vi "testVI.vi"() -> ()   [LabVIEW 2010]
uses:
  <vilib>/Utility/inputDevices.llb/closeJoystick.vi
  C:/Documents and Settings/hakonnod/Desktop/Rotate.llb/rotate 24bit.vi
  <vilib>/picture/picture.llb/Draw True-Color Pixmap.vi
  <vilib>/Utility/inputDevices.llb/joystickAcquire.vi
  <vilib>/picture/3D Picture Control/NI_3D Picture Control.lvlib
panel:
  out "Dial 2":dbl
  in  "Dial":dbl(knob)=4.820308593039098 scale=0.0..10.0
  out "Picture 2":picture
  in  "stop 3":bool
  in  "Pen Color":u32(colorbox)=15671808
  in  "Line Marker":T1={"Width"=1, "Style"=enum."Solid"}
  in  "Rotation Angle (degrees)":dbl=30.0 format="%.2f"
  out "Numeric 5":dbl
  out "Numeric 3":dbl
  out "Numeric 2":dbl
  out "Joystick Info":T2(array[cluster])
  out "Numeric":dbl
  in  "stop 2":bool
  out "Picture":picture
  in  "stop":bool
  out "3D Picture":refnum<vi>(3d-picture)
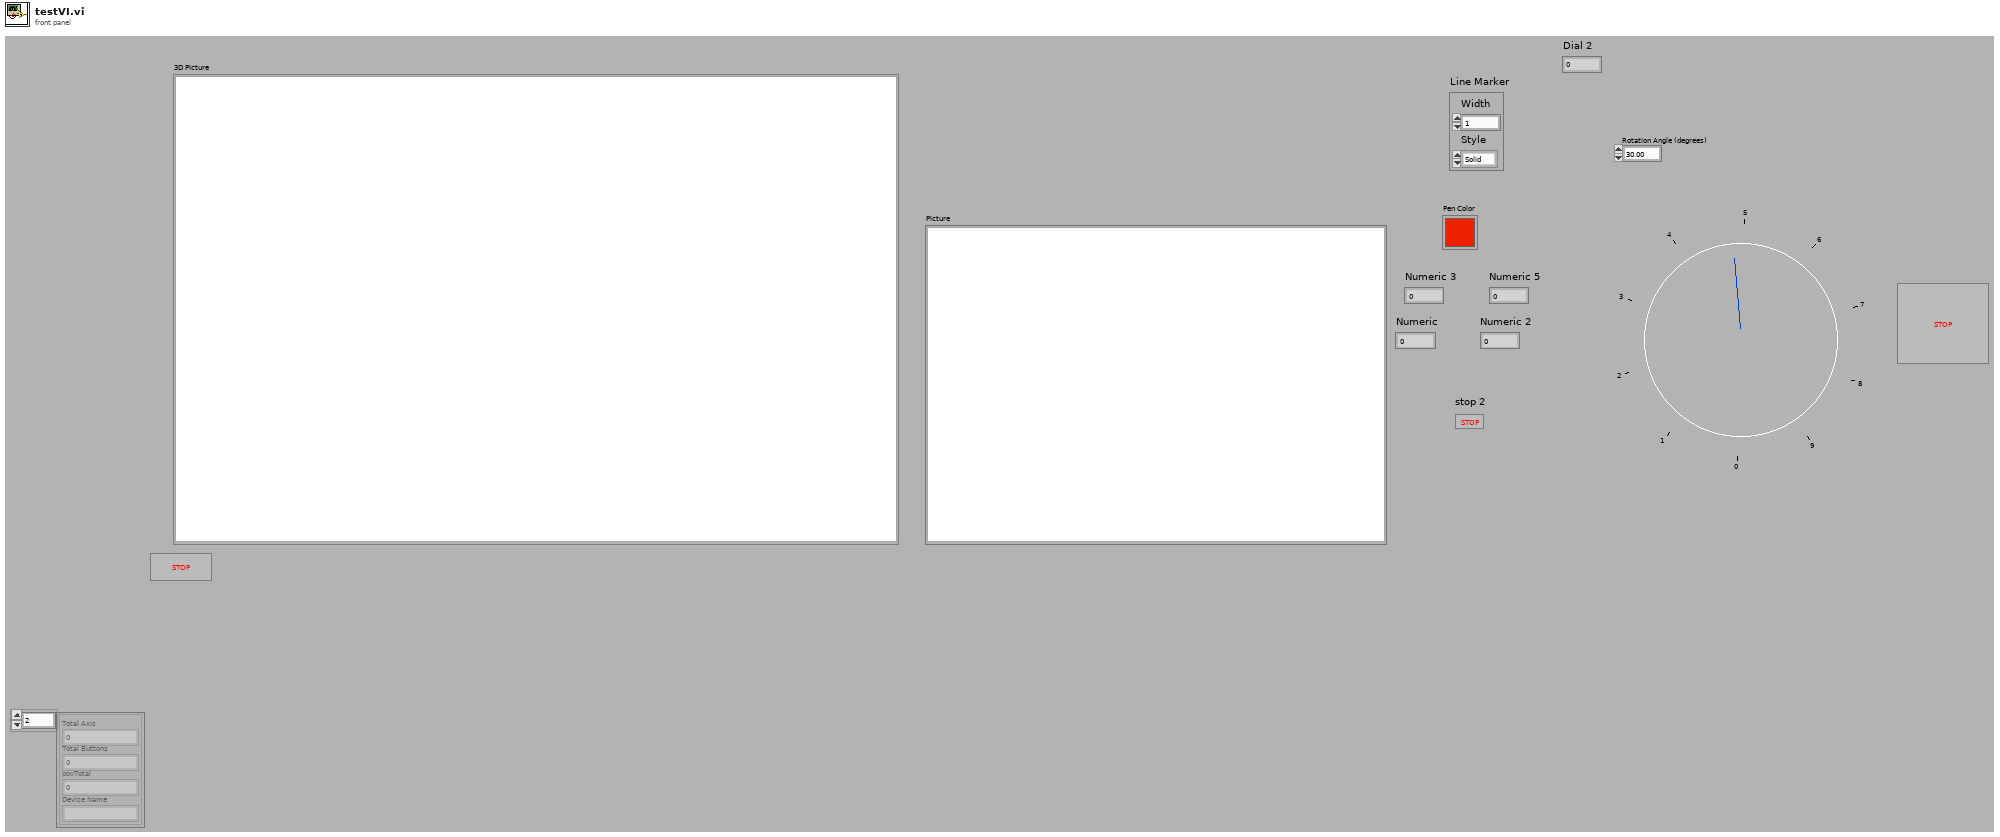
[diagram p1: front panel]
types:
  T1 = cluster{"Width":u16, "Style":enum32{"Solid", "Dash", "Dot", "DashDot", "DashDotDot"}}
  T2 = cluster{"Total Axis":u32, "Total Buttons":u32, "povTotal":u32, "Device Name":string}[]
  T3 = cluster{"Red":sgl, "Green":sgl, "Blue":sgl, "Alpha":sgl}
  T4 = cluster{"axes total":u32, "buttons total":u32, "pov total":u32, "device name":string}[]
  T5 = cluster{"X axis":i32, "Y axis":i32, "Z axis":i32, "X axis rotation":i32, "Y axis rotation":i32, "Z axis rotation":i32, "U axis":i32, "V axis":i32}
  T6 = typedef "imagedata.ctl" = cluster{"image type":i32, "image depth":i32, "image":u8[], "mask":u8[], "colors":u32[], "Rectangle":cluster{"left":i16, "top":i16, "right":i16, "bottom":i16}}
  T7 = typedef "LVMouseTypeDef.ctl" = cluster{"Mouse Position":cluster{"X":i32, "Y":i32}, "Mouse Modifiers":cluster{"Button Down":bool, "Shift Mod":bool, "Menu Mod":bool, "Option Mod":bool}}
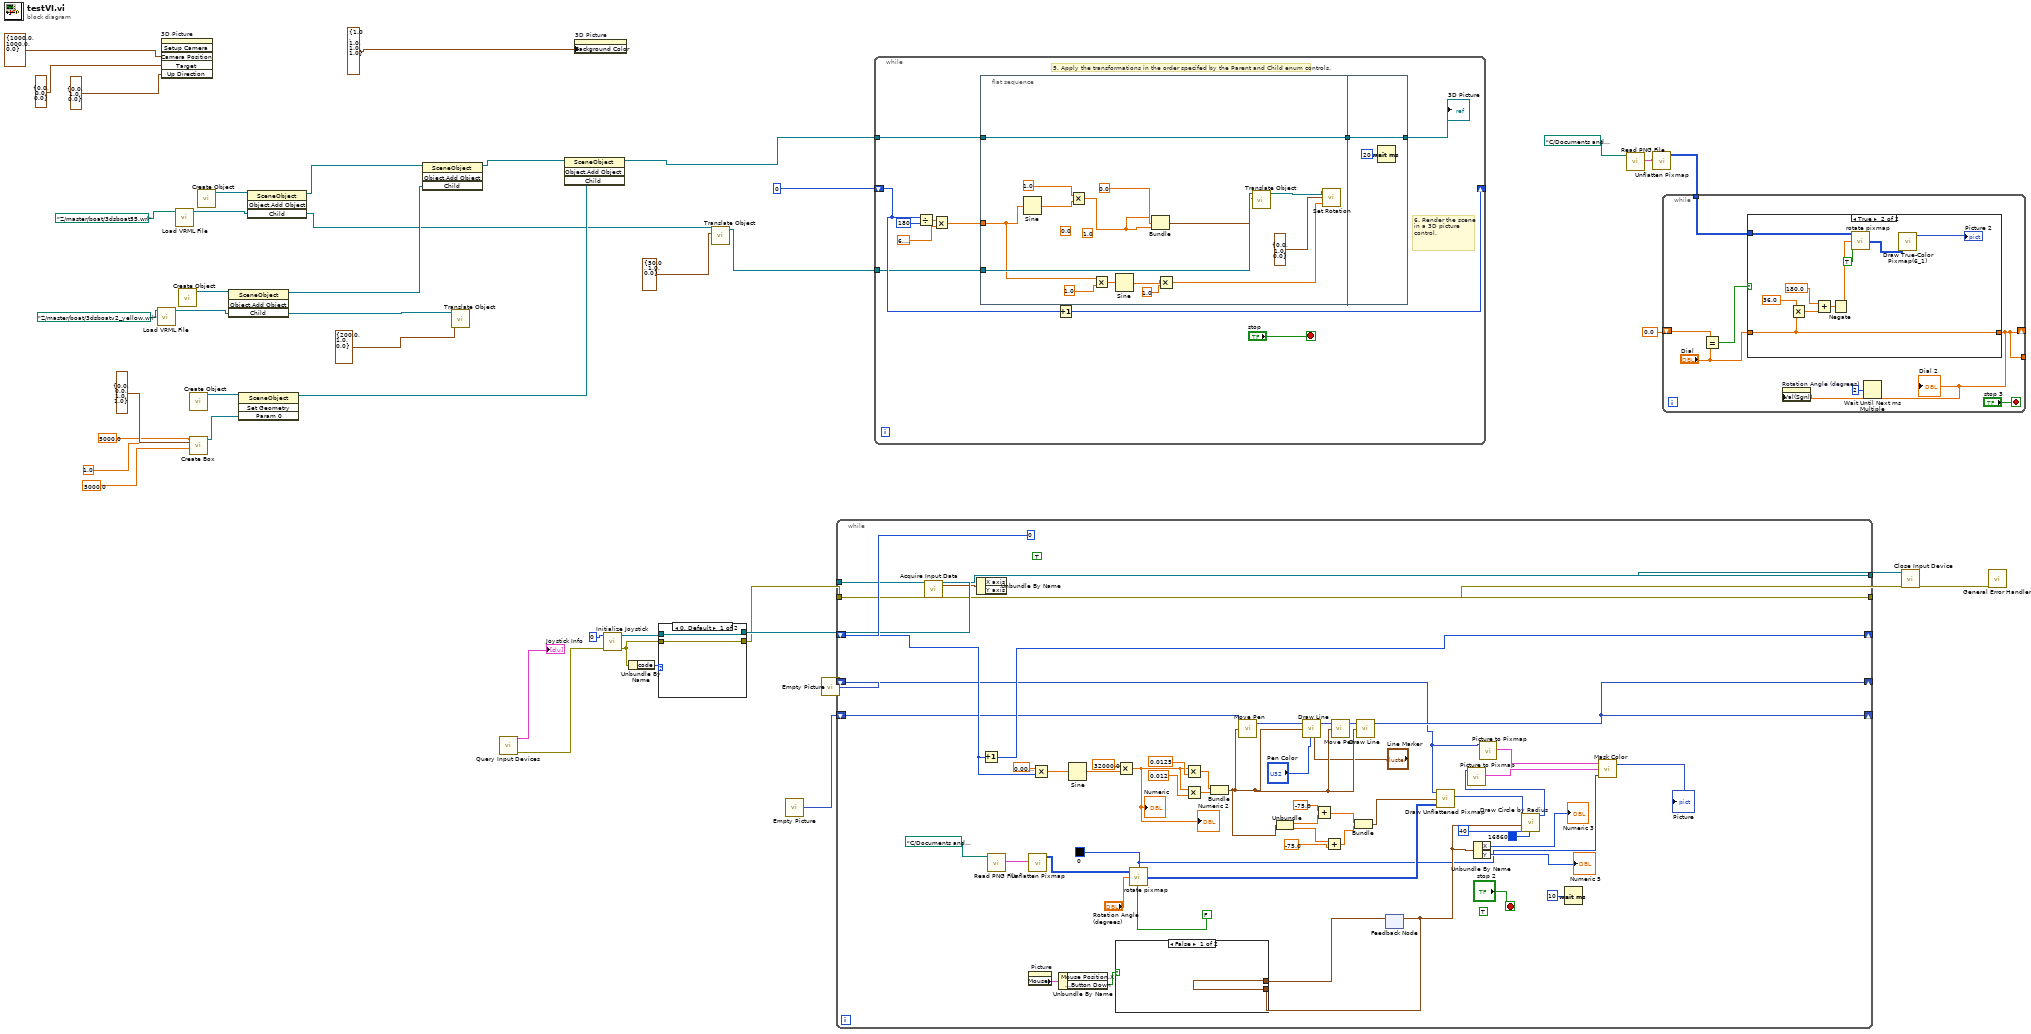
[diagram p0: block diagram]
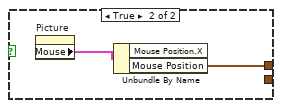
[diagram p4: hidden frame]
diagram:
  (unwired) TRUE
  n1 = call <vilib>:"Load VRML File.vi"("Path"=path "Z:/master/boat/3dsboatv2_yellow.wrl") -> ("Scene:Read Scene File"=w25:refnum<vi>)  [unwired: 9 in, 1 out]
  n2 = invoke on="3D Picture" class="SceneGraphDisp (strict)" method="Setup Camera"("Camera Position"=cluster{"X":sgl, "Y":sgl, "Z":sgl} {"X"=1000.0, "Y"=1000.0, "Z"=0.0}, "Target"=cluster{"X":sgl, "Y":sgl, "Z":sgl} {"X"=0.0, "Y"=0.0, "Z"=0.0} ("Camera Position"), "Up Direction"=cluster{"X":sgl, "Y":sgl, "Z":sgl} {"X"=0.0, "Y"=1.0, "Z"=0.0} ("Camera Position")) -> ()  [unwired: 3 in, 6 out]
  n3 = call <vilib>:"Load VRML File.vi"("Path"=path "Z:/master/boat/3dsboat55.wrl") -> ("Scene:Read Scene File"=w36:refnum<vi>)  [unwired: 9 in, 1 out]
  n4 = call <vilib>:"Create Object.vi"() -> ("Scene:New Object"=w26:refnum<vi>)  [unwired: 10 in, 1 out]
  n5 = call <vilib>:"Create Object.vi"() -> ("Scene:New Object"=w41:refnum<vi>)  [unwired: 10 in, 1 out]
  n6 = call <vilib>:"Create Box.vi"("Color"=T3 {"Red"=0.0, "Green"=0.0, "Blue"=1.0, "Alpha"=1.0}, "Length Z"=sgl 5000.0 ("Red"), "Length Y"=sgl 1.0 ("Red"), "Length X"=sgl 5000.0 ("Red")) -> ("New Box Refnum"=w40:refnum<vi>)  [unwired: 6 in, 1 out]
  n7 = call <vilib>:"Create Object.vi"() -> ("Scene:New Object"=w37:refnum<vi>)  [unwired: 10 in, 1 out]
  n8 = invoke class="SceneObject" method="Object.Add Object"(reference=w26, "Child"=w25) -> (reference out=w20:refnum<vi>, "Child"=w24:refnum<vi>)  [unwired: 2 in, 2 out]
  n9 = invoke class="SceneObject" method="Set Geometry"(reference=w41, "Param 0"=w40) -> (reference out=w28:refnum<vi>)  [unwired: 2 in, 3 out]
  n10 = invoke class="SceneObject" method="Object.Add Object"(reference=w37, "Child"=w36) -> (reference out=w22:refnum<vi>, "Child"=w6:refnum<vi>)  [unwired: 2 in, 2 out]
  n11 = invoke class="SceneObject" method="Object.Add Object"(reference=w22, "Child"=w20) -> (reference out=w21:refnum<vi>)  [unwired: 2 in, 3 out]
  n12 = call <vilib>:"Translate Object.vi"("Translation"=cluster{"X":sgl, "Y":sgl, "Z":sgl} {"X"=200.0, "Y"=1.0, "Z"=0.0} ("Camera Position"), "Scene.Object In"=w24) -> ()  [unwired: 8 in, 2 out]
  n13 = call <vilib>:"Query Input Devices.vi"() -> ("error out"=w18:errorcluster, "joystick info"=→"Joystick Info":T4)  [unwired: 1 in, 9 out]
  n14 = invoke class="SceneObject" method="Object.Add Object"(reference=w21, "Child"=w28) -> (reference out=w29:refnum<vi>)  [unwired: 2 in, 3 out]
  n15 = property on="3D Picture" class="SceneGraphDisp (strict)"("Background Color"=cluster{"X":sgl, "Y":sgl, "Z":sgl, "Z 2":sgl} {"X"=1.0, "Y"=1.0, "Z"=1.0, "Z 2"=1.0} ("Camera Position")) -> ()  [unwired: 2 in, 2 out]
  n16 = call <vilib>:"Initialize Joystick.vi"("error in (no error)"=w18, "device index"=0) -> ("error out"=w13:errorcluster, "device ID"=w14:refnum<k1>)  [unwired: 8 out]
  n17 = Unbundle By Name(w13) -> ("code"=w15:i32)
  n18 = case shown="0, Default" w15 {
    tunnel: w13 -> [w47 w49]
    tunnel: [w47 w49] -> w11
    tunnel: w14 -> [w46 w48]
    tunnel: [w46 w48] -> w12
    frame 0, Default {
    }
    frame -2000000008 {
    }
  }
  n19 = call <vilib>:"Translate Object.vi"("Translation"=cluster{"X":sgl, "Y":sgl, "Z":sgl} {"X"=50.0, "Y"=1.0, "Z"=0.0} ("Camera Position"), "Scene.Object In"=w6) -> ("Scene.Object Out"=w31:refnum<vi>)  [unwired: 8 in, 1 out]
  n20 = call "Empty Picture"() -> ("empty picture"=w5:picture)
  n21 = call "Empty Picture"() -> ("empty picture"=w7:picture)
  n22 = while {
    shift-right: [w103] -> _
    shift-left: 0 -> [w84]
    tunnel: w12 -> [w101]
    tunnel: w11 -> [w100]
    tunnel: [w99] -> w9
    tunnel: [w98] -> w8
    shift-right: [w79] -> _
    shift-left: w7 -> [w56]
    shift-right: [w79] -> _
    shift-left: w5 -> [w80]
    stop <- "stop 2" stop-if-true
    w52 = u32 0 ("Fill Color")
    (unwired) TRUE
    n23 = call-poly <vilib>:"Acquire Input Data.vi"("device ID"=w101, "error in (no error)"=w100) -> ("device ID"=w99:refnum<k1>, "axis info"=w97:T5, "error out"=w98:errorcluster)  [unwired: 15 out]
    n24 = Unbundle By Name(w97) -> ()  [unwired: 2 out]
    n25 = Increment(x=w84) -> (x+1=w103:i32)
    n26 = call <vilib>:"Read PNG File.vi"("path to PNG file"=path "C:/Documents and Settings/hakonnod/My Documents/MATLAB/manualThrusterControl/boat.png") -> ("image data"=w61:T6)  [unwired: 8 in, 2 out]
    n27 = call <vilib>:"Unflatten Pixmap.vi"("image data"=w61) -> ("24-bit pixmap"=w71:u32[][])  [unwired: 4 in, 6 out]
    n28 = property on="Picture" class="Pict"() -> ("Mouse"=w96:T7)  [unwired: 2 in, 2 out]
    n29 = Multiply(x=sgl 0.01 ("Z"), y=w84) -> (x*y=w85:sgl)
    n30 = Unbundle By Name(w96) -> ("Mouse Modifiers.Button Down"=w77:bool)  [unwired: 1 out]
    n31 = Sine(x=w85) -> (sin(x)=w89:sgl)
    n32 = Multiply(x=sgl 32000.0 ("Z"), y=w89) -> (x*y=w88:sgl)
    "Numeric" <- w88
    "Numeric 2" <- w88
    n33 = call-poly "rotate pixmap.vi"("Color Table Index of Fill Color"=w52, "Maintain Center Position?"=FALSE, "Rotation Angle (degrees)"="Rotation Angle (degrees)", "Pixmap"=w71) -> ("Rotated Pixmap"=w62:u32[][])
    n34 = Multiply(x=w88, y=0.0125) -> (x*y=w92:dbl)
    n35 = Multiply(x=w88, y=0.012) -> (x*y=w94:dbl)
    n36 = Bundle(w92, w94) -> (w69:cluster{dbl, dbl})  [unwired: 1 in]
    n37 = call <vilib>:"Move Pen.vi"("new position"=w69, "picture"=w80) -> ("new picture"=w91:picture)  [unwired: 3 in]
    n38 = Unbundle(w69) -> (w64:dbl, w68:dbl)
    n39 = call <vilib>:"Draw Line.vi"("picture"=w91, "end point"=w69, "color(black)"="Pen Color", "pen"="Line Marker") -> ("new picture"=w81:picture)  [unwired: 5 in]
    n40 = Add(x=sgl -75.0 ("X"), y=w64) -> (x+y=w63:dbl)
    n41 = Add(x=w68, y=sgl -75.0 ("X")) -> (x+y=w67:dbl)
    n42 = call <vilib>:"Move Pen.vi"("new position"=w69, "picture"=w81) -> ("new picture"=w82:picture)  [unwired: 3 in]
    n43 = Bundle(w63, w67) -> (w70:cluster{dbl, dbl})  [unwired: 1 in]
    n44 = call <vilib>:"Draw Line.vi"("picture"=w82, "end point"=w69) -> ("new picture"=w79:picture)  [unwired: 7 in]
    n45 = feedback #1() -> (w75:cluster{"X":i32, "Y":i32})  [unwired: 1 in]
    n46 = case shown="False" w77 {
      tunnel: [w104 w105] -> w76
      tunnel: w75 -> [w104 _]
      frame False {
      }
      frame True {
        n47 = property on="Picture" class="Pict"() -> ("Mouse"=w106:T7)  [unwired: 2 in, 2 out]
        n48 = Unbundle By Name(w106) -> ("Mouse Position"=w105:cluster{"X":i32, "Y":i32})  [unwired: 1 out]
      }
    }
    n49 = feedback-in #1(w76) -> ()
    n50 = call-poly <vilib>:"Draw Unflattened Pixmap.vi"("picture"=w56, "top left point(0, 0)"=w70, "data (RGB format)"=w62) -> ("new picture"=w57:picture)  [unwired: 6 in]
    n51 = Unbundle By Name(w75) -> ("X"=→"Numeric 3":i32, "Y"=→"Numeric 5":i32)
    n52 = call <vilib>:"Picture to Pixmap.vi"("picture"=w56) -> ("image data"=w60:T6)  [unwired: 9 in, 1 out]
    n53 = call <vilib>:"Draw Circle by Radius.vi"("color(black)"=u32 16860, "pixel center"=w75, "radius"=40, "picture"=w57) -> ("new picture"=w58:picture)  [unwired: 7 in]
    n54 = call <vilib>:"Picture to Pixmap.vi"("picture"=w58) -> ("image data"=w59:T6)  [unwired: 9 in, 1 out]
    n55 = Wait (ms)(milliseconds to wait=10) -> ()  [unwired: 1 out]
    n56 = call "Mask Color.vi"("Current Mask Color"=w52, "mask data"=w59, "image data"=w60) -> ("Picture"=→"Picture":picture)  [unwired: 1 in]
  }
  n57 = while {
    tunnel: w29 -> [w113]
    shift-right: [w109] -> _
    shift-left: 0 -> [w110]
    tunnel: w31 -> [w108]
    stop <- "stop" stop-if-true
    # "6. Render the scene in a 3D picture control."
    # "5. Apply the transformations in the order specifed by the Parent and Child enum controls."
    n58 = Divide(x=w110, y=180) -> (x/y=w116:dbl)
    n59 = Multiply(x=w116, y=6.283185307179586) -> (x*y=w107:dbl)
    n60 = flat-sequence {
      tunnel: w113 -> [w132]
      tunnel: [w132] -> w112
      tunnel: w107 -> [w125]
      tunnel: w108 -> [w129]
      tunnel: w112 -> [w133]
      tunnel: [w133] -> w111
      frame #0 {
        (unwired) sgl 1.0 ("Z")
        (unwired) sgl 0.0 ("Z")
        n61 = Sine(x=w125) -> (sin(x)=w130:dbl)
        n62 = Multiply(x=sgl 1.0 ("Z"), y=w130) -> (x*y=w126:dbl)
        n63 = Multiply(x=w125, y=sgl 1.0 ("Z")) -> (x*y=w123:dbl)
        n64 = Sine(x=w123) -> (sin(x)=w122:dbl)
        n65 = Bundle(w126, "Z"=sgl 0.0, w126) -> (w128:cluster{dbl, "Z":sgl, dbl})  [unwired: 1 in]
        n66 = Multiply(x=w122, y=sgl 1.0 ("Z")) -> (x*y=w118:dbl)
        n67 = call <vilib>:"Translate Object.vi"("Translation"=w128, "Scene.Object In"=w129) -> ("Scene.Object Out"=w120:refnum<vi>)  [unwired: 8 in, 1 out]
        n68 = call <vilib>:"Set Rotation.vi"("Angle"=w118, "Axis"=cluster{"X":sgl, "Y":sgl, "Z":sgl} {"X"=0.0, "Y"=1.0, "Z"=0.0} ("Camera Position"), "Scene Object"=w120) -> ()  [unwired: 7 in, 2 out]
      }
      frame #1 {
        n69 = Wait (ms)(milliseconds to wait=u32 20) -> ()  [unwired: 1 out]
      }
    }
    n70 = Increment(x=w110) -> (x+1=w109:i32)
    "3D Picture" <- w111
  }
  n71 = call <vilib>:"Read PNG File.vi"("path to PNG file"=path "C:/Documents and Settings/hakonnod/My Documents/MATLAB/manualThrusterControl/boat.png") -> ("image data"=w2:T6)  [unwired: 8 in, 2 out]
  n72 = call <vilib>:"Unflatten Pixmap.vi"("image data"=w2) -> ("24-bit pixmap"=w1:u32[][])  [unwired: 4 in, 6 out]
  n73 = while {
    shift-right: [w135] -> _
    shift-left: 0.0 -> [w141]
    tunnel: w1 -> [w139]
    tunnel: [w135] -> _
    stop <- "stop 3" stop-if-true
    n74 = Equal?(x=w141, y="Dial") -> (x = y?=w140:bool)
    n75 = case shown="True" w140 {
      tunnel: w139 -> [_ w149]
      tunnel: "Dial" -> [w142 w145]
      tunnel: [w142 w145] -> w135
      frame False {
      }
      frame True {
        n76 = Multiply(x=36.0, y=w145) -> (x*y=w151:dbl)
        n77 = Add(x=180.0, y=w151) -> (x+y=w144:dbl)
        n78 = Negate(x=w144) -> (-x=w143:dbl)
        n79 = call-poly "rotate pixmap.vi"("Maintain Center Position?"=TRUE, "Rotation Angle (degrees)"=w143, "Pixmap"=w149) -> ("Rotated Pixmap"=w147:u32[][])  [unwired: 1 in]
        n80 = call <vilib>:"Draw True-Color Pixmap(6_1).vi"("data (RGB format)"=w147) -> ("new picture"=→"Picture 2":picture)  [unwired: 8 in]
      }
    }
    "Dial 2" <- w135
    n81 = property on="Rotation Angle (degrees)" class="DigNum (strict)"("Val(Sgnl)"=w135) -> ()  [unwired: 2 in, 2 out]
    n82 = Wait Until Next ms Multiple(millisecond multiple=u32 2) -> ()  [unwired: 1 out]
  }
  n83 = call-poly <vilib>:"Close Input Device.vi"("error in (no error)"=w8, "device ID"=w9) -> ("error out"=w10:errorcluster)  [unwired: 8 out]
  n84 = call <vilib>:"General Error Handler.vi"("error in (no error)"=w10) -> ()  [unwired: 1 in, 14 out]
